vi "Globals Guided UI.vi"() -> ()   [LabVIEW 2016]
panel:
  out "filename":string
  out "Path":path
  out "Notes":string
  in  "device name: SA0XXXX.YYYYMMDD":string
  in  "project":u16(ring) items=["Quasi-1D chiral proteins", "CZO/STO nanowriting", "Alex Hamilton", "CoO2 nano-sheets", "CoO2 nanoflakes", "TaAs Hall Bar", "Ken Burch 2D Materials on LAOSTO", "Bawendi lead halide nano crystals", "SrIrO3-doped LAO/STO", "Superconductivity in Ti4O7 and \\gamma-Ti3O5 films"]
  in  "Start":bool
  in  "Stop":bool
  in  "user":u16(ring) items=["Shan Hao", "Megan Briggeman", "Aditi Nethwewala", "Dengyue Yang", "Erin Sutton", "Lu Chen", "Yun-Yi Pai", "Yuhe Tang", "Jessica Montone", "Qing Guo", "Joe Albro", "Jianan Li", "Jeremy Levy", "Patrick Irvin"]
  # "1. press to get user names"
  # "2. choose a user"
  # "3. choose a project"
  # "4. choose or type in a\ndevice"
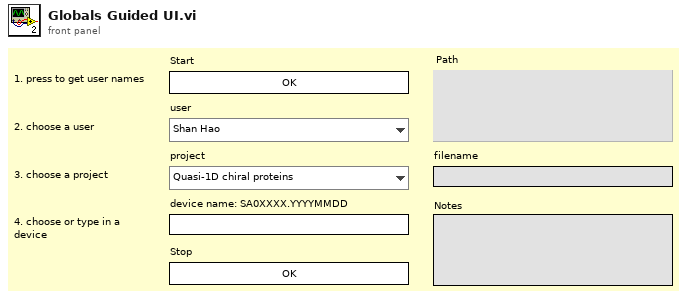
[diagram p1: front panel]
types:
  T1 = enum32{"invalid app kind", "Development System", "Run Time System", "Student Edition", "Embedded LabVIEW", "Evaluation", "Custom"}
  T2 = enum32{"Invalid", "Standard", "Closed", "Hidden", "Minimized", "Maximized"}
  T3 = cluster{"Core":cluster{"Current VI Reference":refnum<vi>, "Close Panel on Exit?":bool}, "Your Boolean data":bool, "user string":string, "research project string":string, "device string":string}
  T4 = cluster{"Current VI Reference":refnum<vi>, "Close Panel on Exit?":bool}
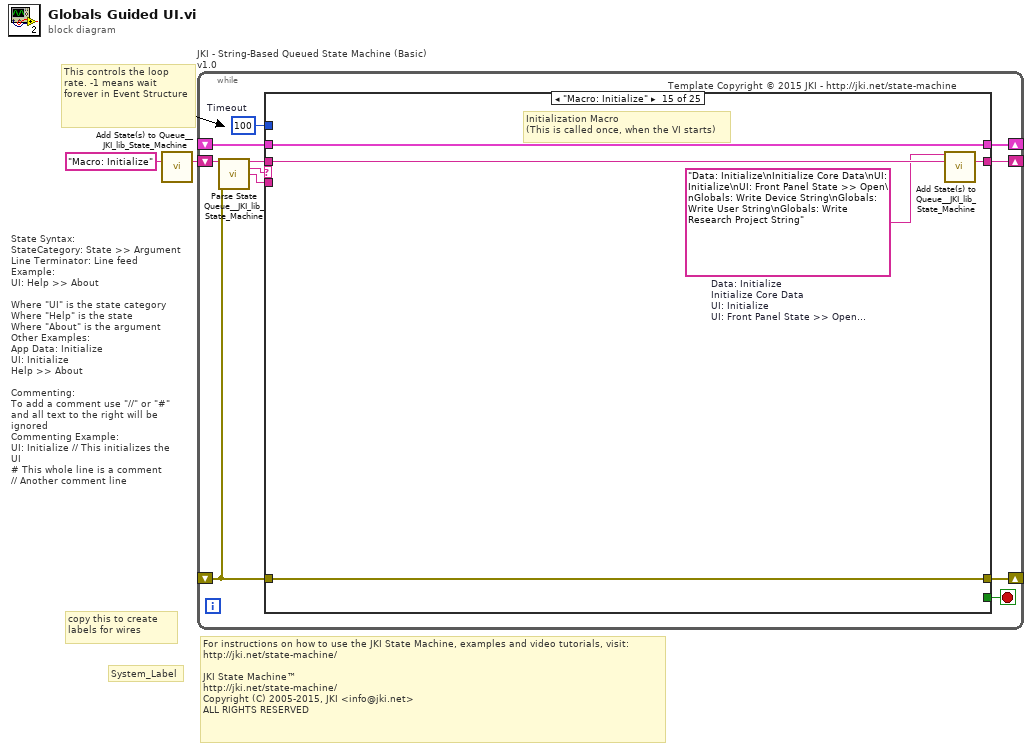
[diagram p0: block diagram]
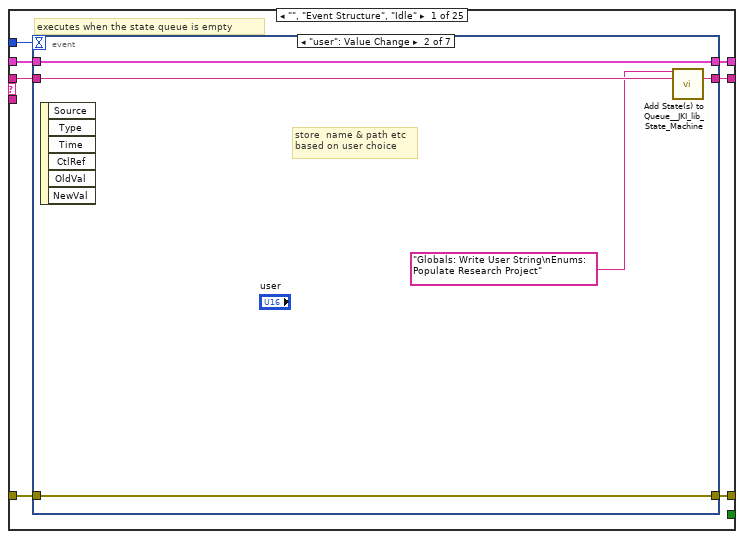
[diagram p2: hidden frame]
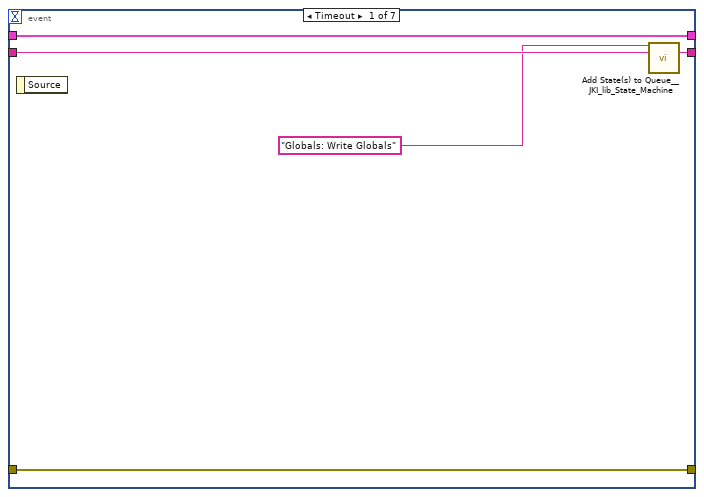
[diagram p3: hidden frame]
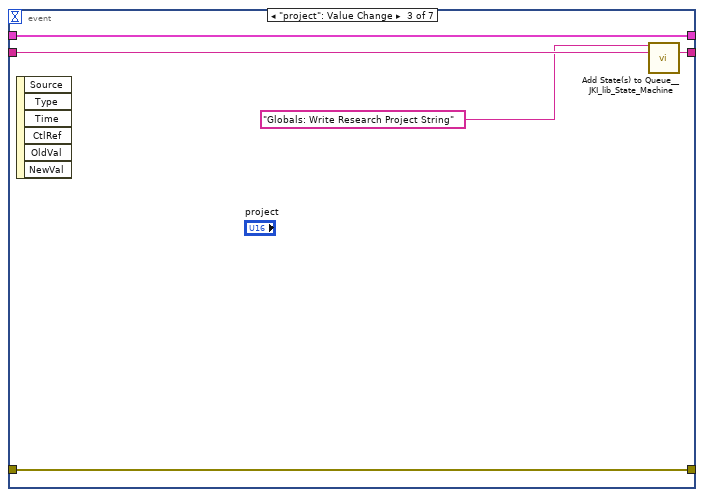
[diagram p4: hidden frame]
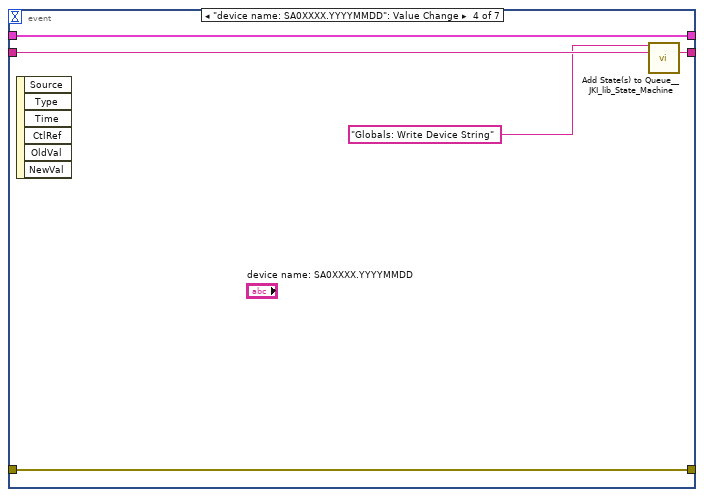
[diagram p5: hidden frame]
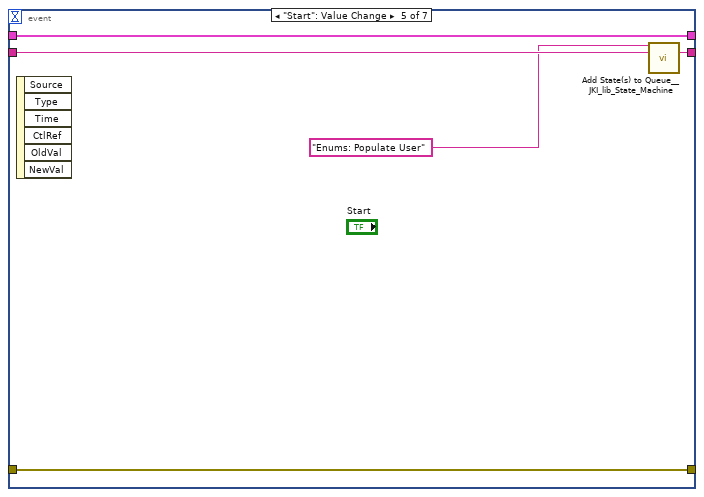
[diagram p6: hidden frame]
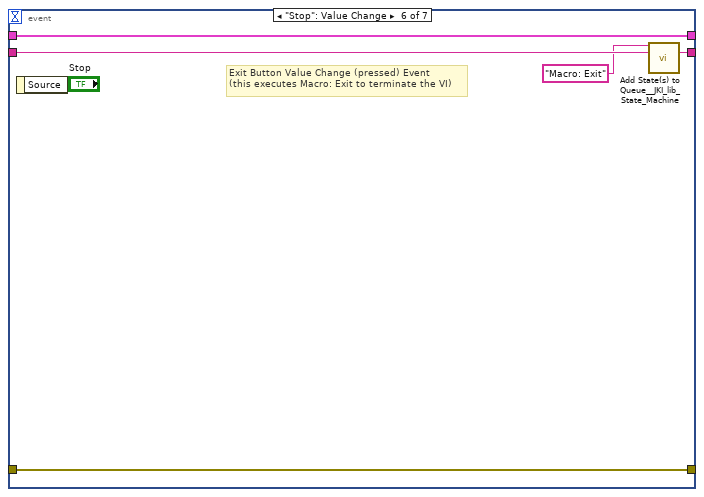
[diagram p7: hidden frame]
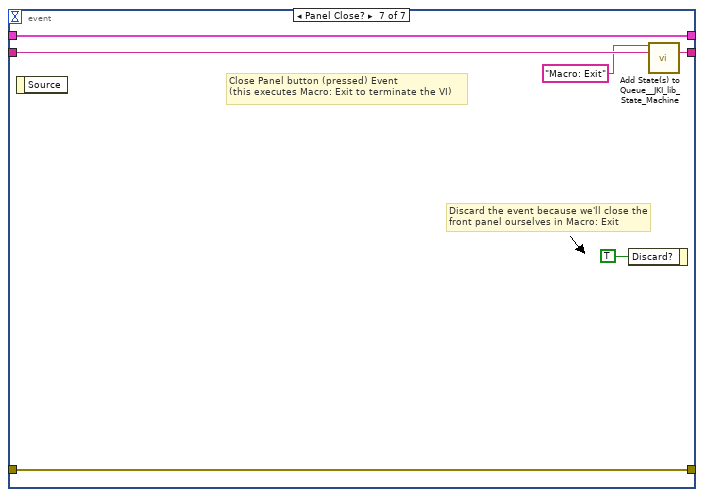
[diagram p8: hidden frame]
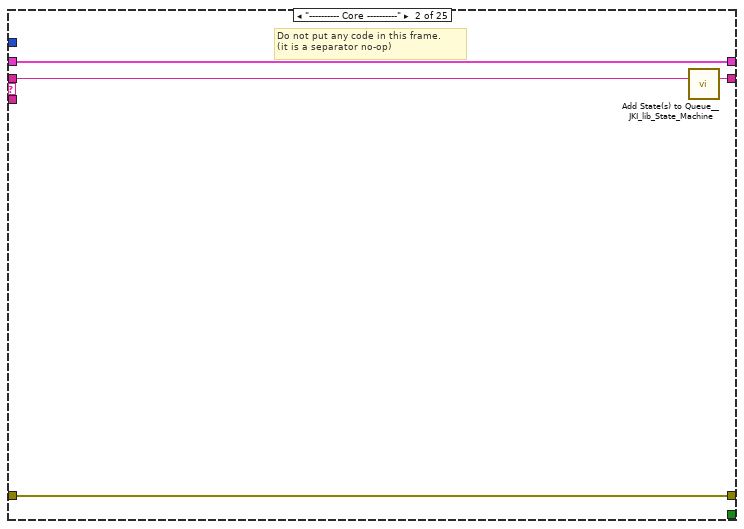
[diagram p9: hidden frame]
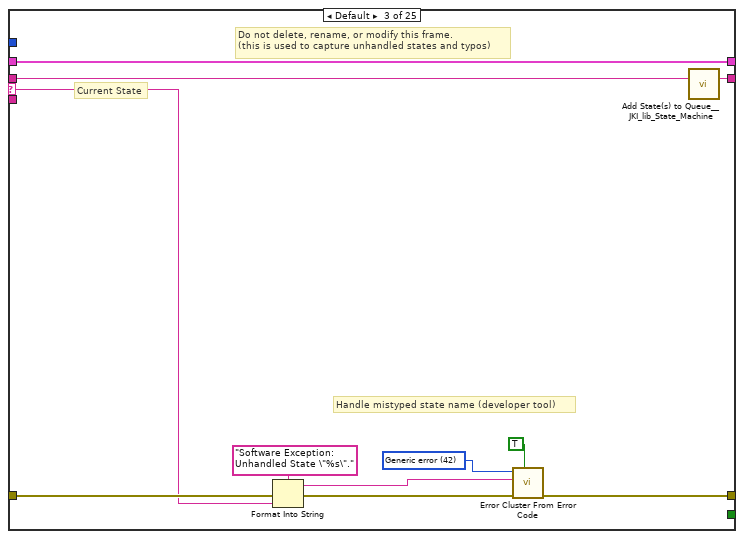
[diagram p10: hidden frame]
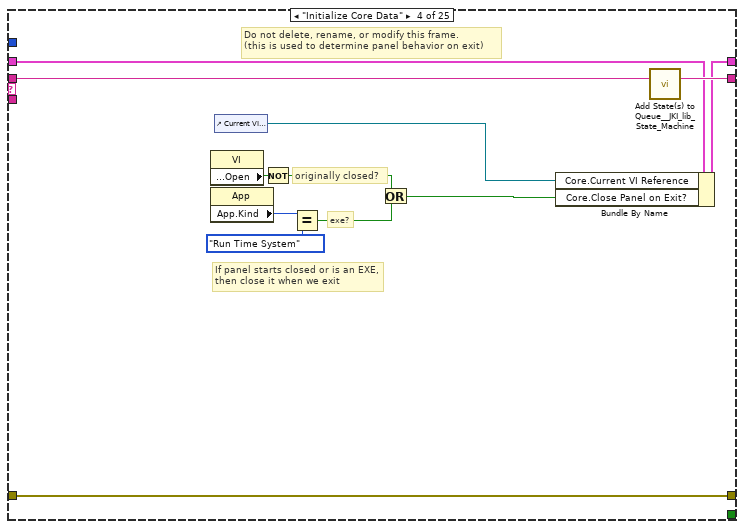
[diagram p11: hidden frame]
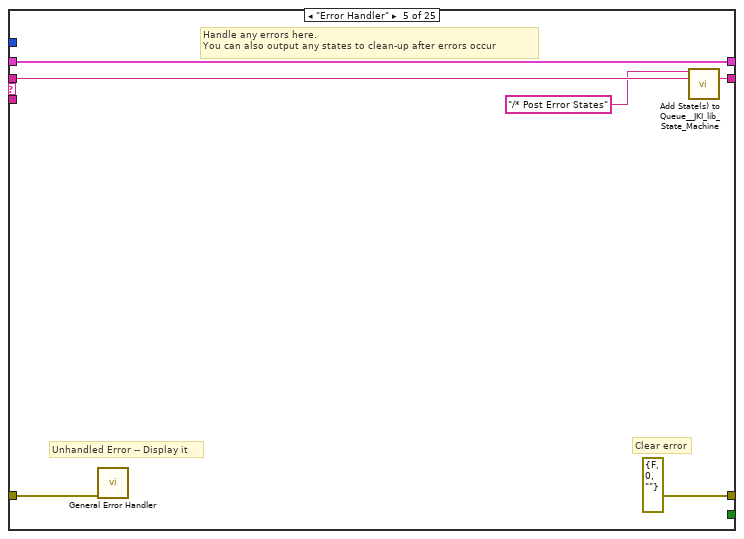
[diagram p12: hidden frame]
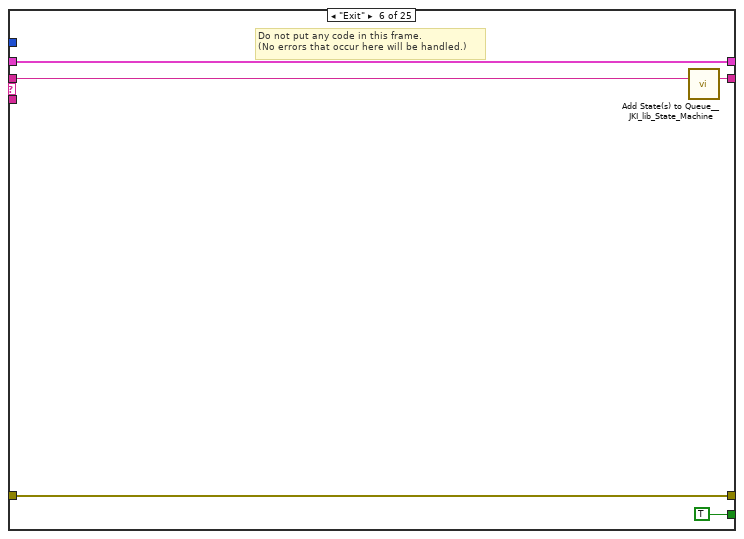
[diagram p13: hidden frame]
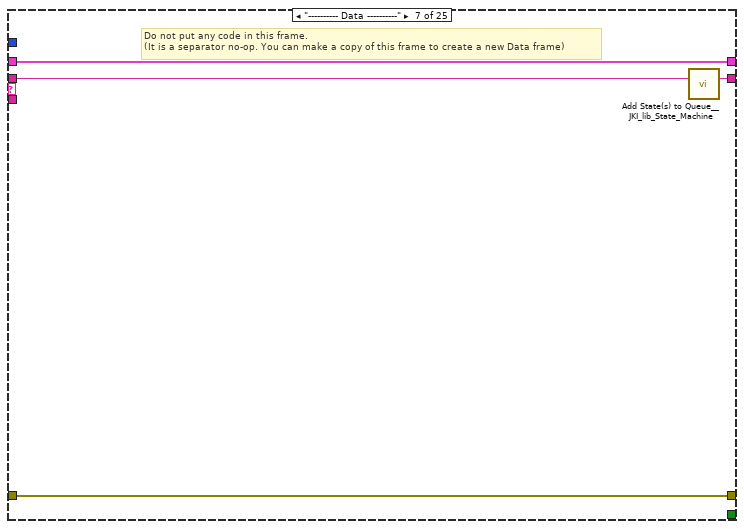
[diagram p14: hidden frame]
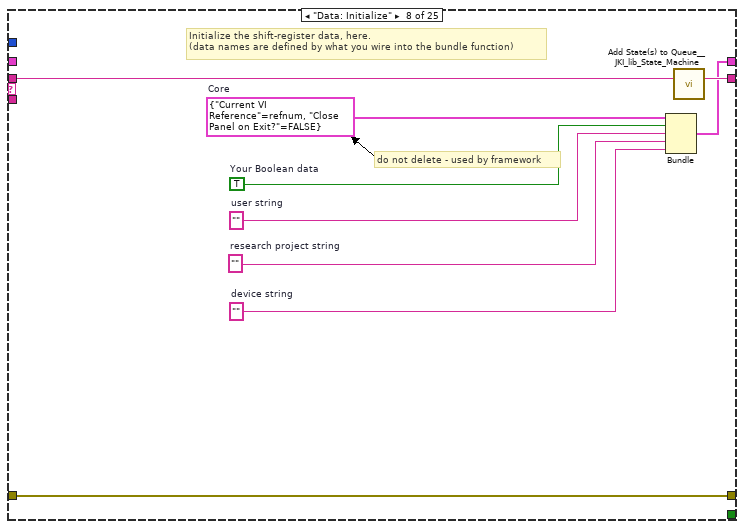
[diagram p15: hidden frame]
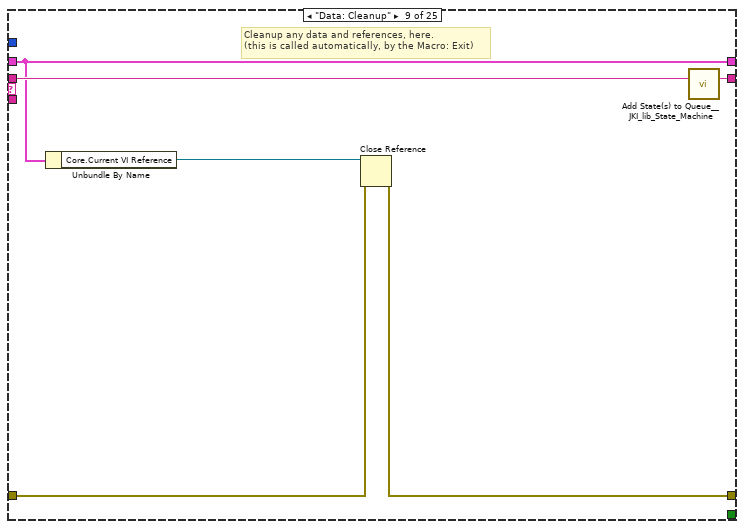
[diagram p16: hidden frame]
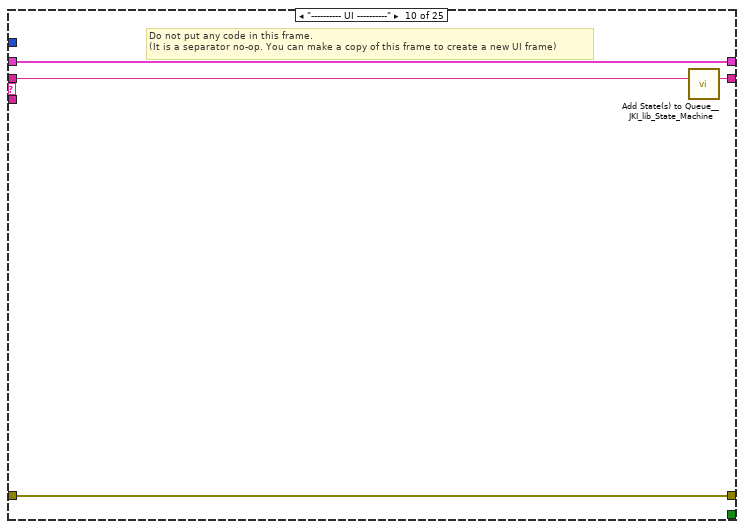
[diagram p17: hidden frame]
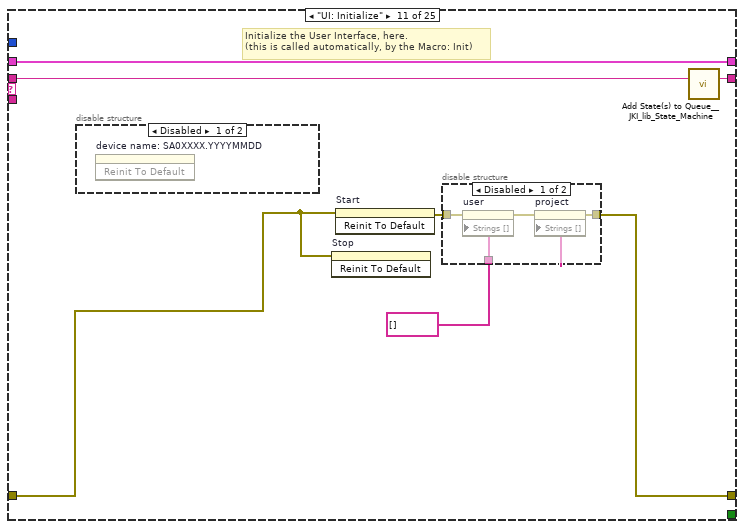
[diagram p18: hidden frame]
diagram:
  # "For instructions on how to use the JKI State Machine, examples and video tutorials, visit:\nhttp://jki.net/state-machine/\n\nJKI State Machine™\nhttp://jki.net/state-machine/\nCopyright (C) 2005-2015, JKI <info@jki.net>\nALL RIGHTS RESERVED"
  # "State Syntax:\nStateCategory: State >> Argument\nLine Terminator: Line feed\nExample:\nUI: Help >> About\n\nWhere \"UI\" is the state category\nWhere \"Help\" is the state\nWhere \"About\" is the argument\nOther Examples:\nApp Data: Initialize\nUI: Initialize\nHelp >> About\n\nCommenting:\nTo add a comment use \"//\" or \"#\" and all text to the right will be ignored\nCommenting Example:\nUI: Initialize // This initializes the UI\n# This whole line is a comment\n// Another comment line"
  # "copy this to create labels for wires"
  # "This controls the loop rate. -1 means wait forever in Event Structure"
  # "System_Label"
  n1 = call <vilib>:"Add State(s) to Queue__JKI_lib_State_Machine.vi"("State(s) in (\"\")"="Macro: Initialize") -> ("States Out"=w2:string)  [unwired: 14 in]
  n2 = while "JKI - String-Based Queued State Machine (Basic) v1.0" {
    shift-right: [w6] -> _
    shift-left: _ -> [w5]
    shift-right: [w9] -> _
    shift-left: _ -> [w3]
    shift-right: [w8] -> _
    shift-left: w2 -> [w10]
    stop <- w7 stop-if-true
    w4 = 100  # Timeout
    # "Template Copyright © 2015 JKI - http://jki.net/state-machine"
    n3 = call <vilib>:"Parse State Queue__JKI_lib_State_Machine.vi"("State Queue"=w10, "Error In (no error)"=w3) -> ("Remaining States"=w12:string, "Current State"=w13:string, "Arguments"=w11:string)  [unwired: 11 in]
    n4 = case shown="\"Macro: Initialize\"" w13 {
      selector: w13 -> [_ _ w61 _ _ _ _ _ _ _ _ _ _ _ _ _ _ _ _ _ _ _ _ _ _]
      tunnel: w12 -> [w20 w60 w65 w83 w89 w94 w98 w107 w113 w117 w124 w134 w145 w171 w176 w186 w190 w195 w204 w209 w218 w224 w230 w236 w250]
      tunnel: w11 -> [_ _ _ _ _ _ _ _ _ _ _ w129 w139 _ _ _ _ _ _ _ _ _ _ _ _]
      tunnel: w5 -> [w18 w57 w63 w74 w86 w92 w95 _ w108 w114 w122 w132 w141 w168 w173 w183 w187 w192 w201 w206 w215 w220 w226 w232 w243]
      tunnel: [w17 w58 w67 w80 errorcluster {"status"=FALSE, "code"=0, "source"=""} ("error out") w91 w96 w104 w109 w115 w119 w130 w142 w169 w174 w184 w188 w193 w202 w207 w216 w222 w228 w234 w248] -> w9
      tunnel: w3 -> [w16 w58 w66 w80 w85 w91 w96 w104 w110 w115 w118 w131 w143 w169 w174 w184 w188 w193 w202 w207 w216 w222 w228 w234 w248]
      tunnel: [w19 w59 w64 w82 w88 w93 w97 w106 w112 w116 w123 w133 w144 w170 w175 w185 w189 w194 w203 w208 w217 w223 w229 w235 w249] -> w8
      tunnel: [_ _ _ _ _ TRUE _ _ _ _ _ _ _ _ _ _ _ _ _ _ _ _ _ _ _] -> w7
      tunnel: [w15 w57 w63 w81 w86 w92 w95 w105 w108 w114 w122 w132 w141 w168 w173 w183 w187 w192 w201 w206 w215 w219 w225 w231 w243] -> w6
      tunnel: w4 -> [w14 _ _ _ _ _ _ _ _ _ _ _ _ _ _ _ _ _ _ _ _ _ _ _ _]
      frame "", "Event Structure", "Idle" {
        # "executes when the state queue is empty"
        n5 = event shown="[1] \"user\": Value Change" {
          selector: _ -> [_ _ _ _ _ _ _]
          dyn-events: _ -> [_ _ _ _ _ _ _]
          timeout: w14 -> [_ _ _ _ _ _ _]
          tunnel: w20 -> [w25 w30 w35 w40 w45 w50 w56]
          tunnel: [w24 w29 w34 w39 w44 w49 w55] -> w19
          tunnel: w18 -> [w22 w26 w32 w37 w42 w47 w53]
          tunnel: [w23 w28 w33 w38 w43 w48 w54] -> w17
          tunnel: w16 -> [w23 w28 w33 w38 w43 w48 w54]
          tunnel: [w22 w26 w32 w37 w42 w47 w53] -> w15
          event Timeout {
            n6 = event-data() -> ()  [unwired: 1 in, 1 out]
            n7 = call <vilib>:"Add State(s) to Queue__JKI_lib_State_Machine.vi"("State(s) in Front (\"\")"="Globals: Write Globals" ("State(s) in Front (\"\")"), "State(s) in (\"\")"=w25) -> ("States Out"=w24:string)  [unwired: 13 in]
          }
          event "user": Value Change {
            # "store  name & path etc\nbased on user choice"
            n8 = event-data() -> ()  [unwired: 1 in, 6 out]
            n9 = call <vilib>:"Add State(s) to Queue__JKI_lib_State_Machine.vi"("State(s) in Front (\"\")"="Globals: Write User String\nEnums: Populate Research Project" ("State(s) in Front (\"\")"), "State(s) in (\"\")"=w30) -> ("States Out"=w29:string)  [unwired: 13 in]
          }
          event "project": Value Change {
            n10 = event-data() -> ()  [unwired: 1 in, 6 out]
            n11 = call <vilib>:"Add State(s) to Queue__JKI_lib_State_Machine.vi"("State(s) in Front (\"\")"="Globals: Write Research Project String" ("State(s) in Front (\"\")"), "State(s) in (\"\")"=w35) -> ("States Out"=w34:string)  [unwired: 13 in]
          }
          event "device name: SA0XXXX.YYYYMMDD": Value Change {
            n12 = event-data() -> ()  [unwired: 1 in, 6 out]
            n13 = call <vilib>:"Add State(s) to Queue__JKI_lib_State_Machine.vi"("State(s) in Front (\"\")"="Globals: Write Device String" ("State(s) in Front (\"\")"), "State(s) in (\"\")"=w40) -> ("States Out"=w39:string)  [unwired: 13 in]
          }
          event "Start": Value Change {
            n14 = event-data() -> ()  [unwired: 1 in, 6 out]
            n15 = call <vilib>:"Add State(s) to Queue__JKI_lib_State_Machine.vi"("State(s) in Front (\"\")"="Enums: Populate User" ("State(s) in Front (\"\")"), "State(s) in (\"\")"=w45) -> ("States Out"=w44:string)  [unwired: 13 in]
          }
          event "Stop": Value Change {
            # "Exit Button Value Change (pressed) Event\n(this executes Macro: Exit to terminate the VI)"
            n16 = event-data() -> ()  [unwired: 1 in, 1 out]
            n17 = call <vilib>:"Add State(s) to Queue__JKI_lib_State_Machine.vi"("State(s) in Front (\"\")"="Macro: Exit", "State(s) in (\"\")"=w50) -> ("States Out"=w49:string)  [unwired: 13 in]
          }
          event Panel Close? {
            # "Discard the event because we'll close the front panel ourselves in Macro: Exit"
            # "Close Panel button (pressed) Event\n(this executes Macro: Exit to terminate the VI)"
            n18 = event-data() -> ()  [unwired: 1 in, 1 out]
            n19 = event-data("Discard?"=TRUE) -> ()  [unwired: 1 in, 1 out]
            n20 = call <vilib>:"Add State(s) to Queue__JKI_lib_State_Machine.vi"("State(s) in Front (\"\")"="Macro: Exit", "State(s) in (\"\")"=w56) -> ("States Out"=w55:string)  [unwired: 13 in]
          }
        }
      }
      frame "---------- Core ----------" {
        # "Do not put any code in this frame.\n(it is a separator no-op)"
        n21 = call <vilib>:"Add State(s) to Queue__JKI_lib_State_Machine.vi"("State(s) in (\"\")"=w60) -> ("States Out"=w59:string)  [unwired: 14 in]
      }
      frame Default {
        w70 = 42 items=["No error", "Argument error", "Memory is full", "Out of zone", "End of file", "File already open", "Generic file I/O error", "File not found", "File permission error", "Disk is full", "Duplicate path", "Too many files open", "System feature not enabled", "Resource file not found", "Cannot add resource", "Resource not found", "Image not found", "Image memory error", "Pen does not exist", "Config type invalid", "Config token not found", "Config parse error", "Config memory error", "Bad external code format", "Bad external code offset", "External code not present", "Null window", "Destroy window error", "Null menu", "Print aborted", "Bad print record", "Print driver error", "Windows error during printing", "Memory error during printing", "Print dialog error", "Generic print error", "Invalid device refnum", "Device not found", "Device parameter error", "Device unit error", "Cannot open device", "Device call aborted", "Generic error", "Cancelled by user", "Object ID too low", "Object ID too high", "Object not in heap", "Unknown heap", "Unknown object (invalid DefProc)", "Unknown object (DefProc not in table)", "Message out of range", "Invalid (null) method", "Unknown message", "Manager call not supported", "Bad address", "Network operation in progress", "Network operation timed out", "Connection is busy", "Network attribute not supported", "Network error", "Address in use", "System out of memory", "Connection aborted", "Connection refused", "Not connected", "Already connected", "Connection closed", "Initialization error (interapplication manager)", "Bad occurrence", "Wait on unbound occurrence handler", "Occurrence queue overflow", "Datalog type conflict", "Unused", "Unrecognized type (interapplication manager)", "Memory corrupt", "Failed to make temporary DLL", "Old CIN version", "Drag socket not found", "Failed to load drop-object", "Failed to register OLE object", "Failed to release OLE object", "Format specifier type mismatch", "Unknown format specifier", "Too few format specifiers", "Too many format specifiers", "Scan failed", "Newer CIN version", "Error converting to variant", "Runtime menu error", "Password tampered", "Variant attribute not found", "Incompatible variant data type", "Event data is not available", "Event Store is not present", "Occurrence is not found", "Event Queue is not created", "Event info is not available", "Refnum passed is NULL", "Error retrieving Class GUID", "Error retrieving CoClass GUID", "Error retrieving TypeLib GUID.", "Bad built application magic bytes.", "Specific driver is different from the specific driver associated with the Logical Name.", "There is no session opened to the class driver.", "Max Error", "MAX - Error with config objects", "MAX - Error loading configuration", "MAX - Group not supported"]
        # "Current State"
        # "Do not delete, rename, or modify this frame.\n(this is used to capture unhandled states and typos)"
        # "Handle mistyped state name (developer tool)"
        n22 = Format Into String(format string="Software Exception: Unhandled State \"%s\"." ("message"), error in=w66, w61) -> (resulting string=w69:string, error out=w68:errorcluster)  [unwired: 1 in]
        n23 = call <vilib>:"Error Cluster From Error Code.vi"("show call chain? (False)"=TRUE, "error in (no error)"=w68, "error message (\"\")"=w69, "error code (0)"=w70) -> ("error out"=w67:errorcluster)  [unwired: 5 in]
        n24 = call <vilib>:"Add State(s) to Queue__JKI_lib_State_Machine.vi"("State(s) in (\"\")"=w65) -> ("States Out"=w64:string)  [unwired: 14 in]
      }
      frame "Initialize Core Data" {
        # "Do not delete, rename, or modify this frame.\n(this is used to determine panel behavior on exit)"
        # "originally closed?"
        # "exe?"
        # "If panel starts closed or is an EXE, then close it when we exit"
        n25 = property class="VI"() -> ("Front Panel.Open"=w79:bool)  [unwired: 2 in, 2 out]
        n26 = property class="App"() -> ("App.Kind"=w78:T1)  [unwired: 2 in, 2 out]
        n27 = control-ref of="Current VI Reference"() -> (w72:refnum<vi>)
        n28 = Not(x=w79) -> (.not. x?=w76:bool)
        n29 = Equal?(x=w78, y=T1."Run Time System" ("Application:Kind")) -> (x = y?=w75:bool)
        n30 = Or(x=w76, y=w75) -> (x .or. y?=w73:bool)
        n31 = Bundle By Name(cluster=w74, "Core.Current VI Reference"=w72, "Core.Close Panel on Exit?"=w73) -> (w81:T3)
        n32 = call <vilib>:"Add State(s) to Queue__JKI_lib_State_Machine.vi"("State(s) in (\"\")"=w83) -> ("States Out"=w82:string)  [unwired: 14 in]
      }
      frame "Error Handler" {
        # "Unhandled Error -- Display it"
        # "Handle any errors here.\nYou can also output any states to clean-up after errors occur"
        # "Clear error"
        n33 = call <vilib>:"General Error Handler.vi"("error in (no error)"=w85) -> ()  [unwired: 10 in, 5 out]
        n34 = call <vilib>:"Add State(s) to Queue__JKI_lib_State_Machine.vi"("State(s) in Front (\"\")"="/* Post Error States", "State(s) in (\"\")"=w89) -> ("States Out"=w88:string)  [unwired: 13 in]
      }
      frame "Exit" {
        # "Do not put any code in this frame.\n(No errors that occur here will be handled.)"
        n35 = call <vilib>:"Add State(s) to Queue__JKI_lib_State_Machine.vi"("State(s) in (\"\")"=w94) -> ("States Out"=w93:string)  [unwired: 14 in]
      }
      frame "---------- Data ----------" {
        # "Do not put any code in this frame.\n(It is a separator no-op. You can make a copy of this frame to create a new Data frame)"
        n36 = call <vilib>:"Add State(s) to Queue__JKI_lib_State_Machine.vi"("State(s) in (\"\")"=w98) -> ("States Out"=w97:string)  [unwired: 14 in]
      }
      frame "Data: Initialize" {
        w99 = ""  # device string
        w100 = ""  # research project string
        w101 = T4 {"Current VI Reference"=refnum, "Close Panel on Exit?"=FALSE}  # Core
        w103 = TRUE  # Your Boolean data
        w102 = ""  # user string
        # "do not delete - used by framework"
        # "Initialize the shift-register data, here.\n(data names are defined by what you wire into the bundle function)"
        n37 = Bundle("Core"=w101, "Your Boolean data"=w103, "user string"=w102, "research project string"=w100, "device string"=w99) -> (w105:T3)  [unwired: 1 in]
        n38 = call <vilib>:"Add State(s) to Queue__JKI_lib_State_Machine.vi"("State(s) in (\"\")"=w107) -> ("States Out"=w106:string)  [unwired: 14 in]
      }
      frame "Data: Cleanup" {
        # "Cleanup any data and references, here.\n(this is called automatically, by the Macro: Exit)"
        n39 = Unbundle By Name(w108) -> ("Core.Current VI Reference"=w111:refnum<vi>)
        n40 = Close Reference(reference=w111, error in (no error)=w110) -> (error out=w109:errorcluster)
        n41 = call <vilib>:"Add State(s) to Queue__JKI_lib_State_Machine.vi"("State(s) in (\"\")"=w113) -> ("States Out"=w112:string)  [unwired: 14 in]
      }
      frame "---------- UI ----------" {
        # "Do not put any code in this frame.\n(It is a separator no-op. You can make a copy of this frame to create a new UI frame)"
        n42 = call <vilib>:"Add State(s) to Queue__JKI_lib_State_Machine.vi"("State(s) in (\"\")"=w117) -> ("States Out"=w116:string)  [unwired: 14 in]
      }
      frame "UI: Initialize" {
        # "Initialize the User Interface, here.\n(this is called automatically, by the Macro: Init)"
        n43 = disable-structure shown="Disabled" {
          frame Disabled {
            n44 = invoke on="device name: SA0XXXX.YYYYMMDD" class="Str" method="Reinit To Default"() -> ()  [unwired: 3 in, 3 out]
          }
          frame Enabled {
          }
        }
        n45 = invoke on="Stop" class="Bool" method="Reinit To Default"(error in=w118) -> ()  [unwired: 2 in, 3 out]
        n46 = invoke on="Start" class="Bool" method="Reinit To Default"(error in=w118) -> (error out=w121:errorcluster)  [unwired: 2 in, 2 out]
        n47 = disable-structure shown="Disabled" {
          disable-tunnel: w121 -> [w127 _]
          disable-tunnel: string[] [] ("Strings []") -> [w126 _]
          disable-tunnel: [w125 _] -> w119
          frame Disabled {
            n48 = property on="user" class="Ring (strict)"(error in=w127, "Strings []"=w126) -> (error out=w128:errorcluster)  [unwired: 1 in, 1 out]
            n49 = property on="project" class="Ring (strict)"(error in=w128, "Strings []"=w126) -> (error out=w125:errorcluster)  [unwired: 1 in, 1 out]
          }
          frame Enabled {
          }
        }
        n50 = call <vilib>:"Add State(s) to Queue__JKI_lib_State_Machine.vi"("State(s) in (\"\")"=w124) -> ("States Out"=w123:string)  [unwired: 14 in]
      }
      frame "UI: Cursor Set" {
        # "Argument"
        # "Set and Unset Cursor Busy.\n(Usage: \"UI: Cursor Set >> Busy|Idle\")"
        n51 = case shown="\"Idle\", Default" w129 {
          tunnel: w131 -> [w136 w138]
          tunnel: [w135 w137] -> w130
          frame "Idle", Default {
            n52 = call <vilib>:"Unset Busy.vi"("error in (no error)"=w136) -> ("error out"=w135:errorcluster)  [unwired: 10 in]
          }
          frame "Busy" {
            n53 = call <vilib>:"Set Busy.vi"("error in (no error)"=w138) -> ("error out"=w137:errorcluster)  [unwired: 9 in, 1 out]
          }
        }
        n54 = call <vilib>:"Add State(s) to Queue__JKI_lib_State_Machine.vi"("State(s) in (\"\")"=w134) -> ("States Out"=w133:string)  [unwired: 14 in]
      }
      frame "UI: Front Panel State" {
        # "Argument"
        # "Set Front Panel Open or Closed\n(Usage: \"UI: Front Panel State >> Open|Close\")"
        n55 = Unbundle By Name(w141) -> ("Core.Current VI Reference"=w140:refnum<vi>)
        n56 = case shown="\"Open\", Default" w139 {
          tunnel: w143 -> [w149 w162]
          tunnel: [w151 w163] -> w142
          tunnel: w140 -> [w150 w160]
          frame "Open", Default {
            n57 = property class="VI"(reference=w150, error in=w149) -> (reference out=w147:refnum<vi>, error out=w148:errorcluster, "Front Panel.Open"=w146:bool)
            n58 = case shown="False" w146 {
              tunnel: [w154 w157] -> w151
              tunnel: w148 -> [w153 w157]
              tunnel: w147 -> [w152 _]
              frame False {
                n59 = invoke class="VI" method="FP.Open"(reference=w152, error in=w153, "Activate"=TRUE, "State"=T2."Standard") -> (error out=w154:errorcluster)  [unwired: 1 in, 4 out]
              }
              frame True {
              }
            }
          }
          frame "Close" {
            n60 = property class="VI"(reference=w160, error in=w162) -> (reference out=w159:refnum<vi>, error out=w161:errorcluster, "Front Panel.Open"=w158:bool)
            n61 = case shown="True" w158 {
              tunnel: [w164 w167] -> w163
              tunnel: w161 -> [w164 w166]
              tunnel: w159 -> [_ w165]
              frame False {
              }
              frame True {
                n62 = invoke class="VI" method="FP.Close"(reference=w165, error in=w166) -> (error out=w167:errorcluster)  [unwired: 1 in, 2 out]
              }
            }
          }
        }
        n63 = call <vilib>:"Add State(s) to Queue__JKI_lib_State_Machine.vi"("State(s) in (\"\")"=w145) -> ("States Out"=w144:string)  [unwired: 14 in]
      }
      frame "---------- Macro ----------" {
        # "Do not put any code in this frame.\n(It is a separator no-op. You can make a copy of this frame to create a new Macro frame)"
        n64 = call <vilib>:"Add State(s) to Queue__JKI_lib_State_Machine.vi"("State(s) in (\"\")"=w171) -> ("States Out"=w170:string)  [unwired: 14 in]
      }
      frame "Macro: Initialize" {
        w172 = "Data: Initialize\nInitialize Core Data\nUI: Initialize\nUI: Front Panel State >> Open\nGlobals: Write Device String\nGlobals: Write User String\nGlobals: Write Research Project String"  # Data: Initialize Initialize Core Data UI: Initialize UI: Front Panel State >> Open Globals: Write Device String Globals: Write User String Globals: Write Research Project String
        # "Initialization Macro\n(This is called once, when the VI starts)"
        n65 = call <vilib>:"Add State(s) to Queue__JKI_lib_State_Machine.vi"("State(s) in Front (\"\")"=w172, "State(s) in (\"\")"=w176) -> ("States Out"=w175:string)  [unwired: 13 in]
      }
      frame "Macro: Exit" {
        # "Exit Macro\n(This is called once, when the VI exits)"
        n66 = Unbundle By Name(w183) -> ("Core.Close Panel on Exit?"=w182:bool)
        n67 = Select(t="Enums: Write Notes\nUI: Front Panel State >> Close", s=w182, f="") -> (s? t:f=w179:string)
        n68 = call <vilib>:"Add State(s) to Queue__JKI_lib_State_Machine.vi"("State(s) in (\"\")"=w179, "State(s) at Back (\"\")"="Data: Cleanup\nExit") -> ("States Out"=w177:string)  [unwired: 13 in]
        n69 = call <vilib>:"Add State(s) to Queue__JKI_lib_State_Machine.vi"("State(s) in Front (\"\")"=w177, "State(s) in (\"\")"=w186) -> ("States Out"=w185:string)  [unwired: 13 in]
      }
      frame "---------- Enums ----------" {
        # "Template Separator\n(You can make a copy of, or modify, this frame)"
        n70 = call <vilib>:"Add State(s) to Queue__JKI_lib_State_Machine.vi"("State(s) in (\"\")"=w190) -> ("States Out"=w189:string)  [unwired: 14 in]
      }
      frame "Enums: Populate User" {
        n71 = flat-sequence {
          tunnel: [w196] -> w191
          frame #0 {
            # "this code represents call to asana asking for users"
            n72 = Spreadsheet String To Array(delimiter (Tab)="\n", format string="%s", spreadsheet string="Shan Hao\nMegan Briggeman\nAditi Nethwewala\nDengyue Yang\nErin Sutton\nLu Chen\nYun-Yi Pai\nYuhe Tang\nJessica Montone\nQing Guo\nJoe Albro\nJianan Li\nJeremy Levy\nPatrick Irvin", array type (2D Dbl)=string[] []) -> (array=w196:string[])
          }
        }
        n73 = property on="user" class="Ring (strict)"("Strings []"=w191) -> ()  [unwired: 2 in, 2 out]
        n74 = call <vilib>:"Add State(s) to Queue__JKI_lib_State_Machine.vi"("State(s) in (\"\")"=w195) -> ("States Out"=w194:string)  [unwired: 14 in]
      }
      frame "Enums: Populate Sample" {
        n75 = call <vilib>:"Add State(s) to Queue__JKI_lib_State_Machine.vi"("State(s) in (\"\")"=w204) -> ("States Out"=w203:string)  [unwired: 14 in]
      }
      frame "Enums: Populate Research Project" {
        n76 = flat-sequence {
          tunnel: [w210] -> w205
          frame #0 {
            # "this code represents call to asana asking for research project names"
            n77 = Spreadsheet String To Array(delimiter (Tab)="\n", format string="%s", spreadsheet string="Quasi-1D chiral proteins\nCZO/STO nanowriting\nAlex Hamilton\nCoO2 nano-sheets\nCoO2 nanoflakes\nTaAs Hall Bar\nKen Burch 2D Materials on LAOSTO\nBawendi lead halide nano crystals\nSrIrO3-doped LAO/STO\nSuperconductivity in Ti4O7 and \\gamma-Ti3O5 films", array type (2D Dbl)=string[] []) -> (array=w210:string[])
          }
        }
        n78 = property on="project" class="Ring (strict)"("Strings []"=w205) -> ()  [unwired: 2 in, 2 out]
        n79 = call <vilib>:"Add State(s) to Queue__JKI_lib_State_Machine.vi"("State(s) in (\"\")"=w209) -> ("States Out"=w208:string)  [unwired: 14 in]
      }
      frame "---------- Globals ----------" {
        # "Template Separator\n(You can make a copy of, or modify, this frame)"
        n80 = call <vilib>:"Add State(s) to Queue__JKI_lib_State_Machine.vi"("State(s) in (\"\")"=w218) -> ("States Out"=w217:string)  [unwired: 14 in]
      }
      frame "Globals: Write Device String" {
        n81 = property on="device name: SA0XXXX.YYYYMMDD" class="Str"() -> ("Text.Text"=w221:string)  [unwired: 2 in, 2 out]
        n82 = Bundle By Name(cluster=w220, "device string"=w221) -> (w219:T3)
        n83 = call <vilib>:"Add State(s) to Queue__JKI_lib_State_Machine.vi"("State(s) in (\"\")"=w224) -> ("States Out"=w223:string)  [unwired: 14 in]
      }
      frame "Globals: Write User String" {
        n84 = property on="user" class="Ring (strict)"() -> ("RingText.Text"=w227:string)  [unwired: 2 in, 2 out]
        n85 = Bundle By Name(cluster=w226, "user string"=w227) -> (w225:T3)
        n86 = call <vilib>:"Add State(s) to Queue__JKI_lib_State_Machine.vi"("State(s) in (\"\")"=w230) -> ("States Out"=w229:string)  [unwired: 14 in]
      }
      frame "Globals: Write Research Project String" {
        n87 = property on="project" class="Ring (strict)"() -> ("RingText.Text"=w233:string)  [unwired: 2 in, 2 out]
        n88 = Bundle By Name(cluster=w232, "research project string"=w233) -> (w231:T3)
        n89 = call <vilib>:"Add State(s) to Queue__JKI_lib_State_Machine.vi"("State(s) in (\"\")"=w236) -> ("States Out"=w235:string)  [unwired: 14 in]
      }
      frame "Globals: Write Globals" {
        n90 = Unbundle By Name(w243) -> ("user string"=w237:string, "research project string"=w239:string, "device string"=w238:string)
        "filename" <- w238
        n91 = Build Array(w238, w239, w237) -> (w247:string[])
        n92 = Array To Spreadsheet String(delimiter (Tab)="\n", array=w247, 3:"%s" ("format string")) -> (spreadsheet string=→"Notes":string)
        n93 = Build Path(base path=path "G:/Team Drives/LevyLabData" ("Path"), name or relative path=w239) -> (appended path=w240:path)
        n94 = Build Path(base path=w240, name or relative path=w238) -> (appended path=→"Path":path)
        n95 = call <vilib>:"Add State(s) to Queue__JKI_lib_State_Machine.vi"("State(s) in (\"\")"=w250) -> ("States Out"=w249:string)  [unwired: 14 in]
      }
    }
  }
